vi "Read UUT_Pedigree.vi"(8 "error in (no error)":errorcluster, 11 "Instruments in":refnum<class "Instruments.lvclass">) -> (0 "error out":errorcluster, 2 "Pedigree":enum16{"STAT", "BB", "PT", "EM", "FT"}(ring), 3 "Instruments out":refnum<class "Instruments.lvclass">)   [LabVIEW 2019, in "Instruments.lvlib" / "Instruments.lvclass"]
uses:
  Library/Instruments.lvclass
  Library/Instruments.lvclass/Instruments.ctl
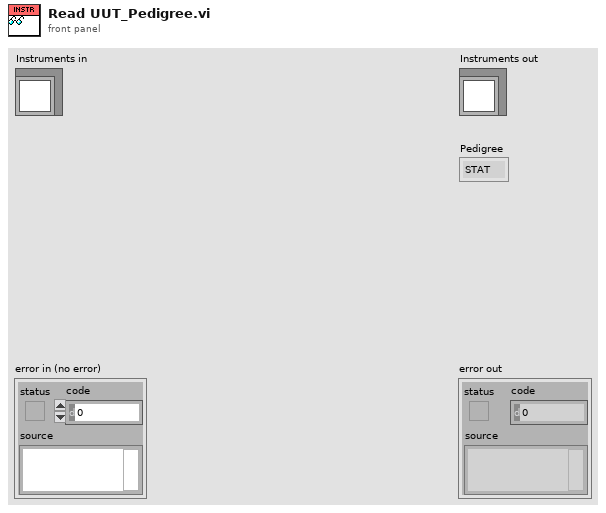
[diagram p1: front panel]
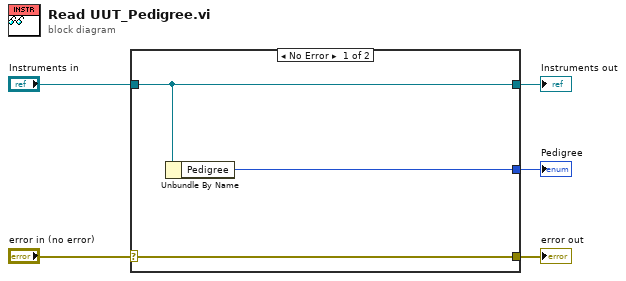
[diagram p0: block diagram]
diagram:
  n1 = case shown="No Error" "error in (no error)" {
    selector: "error in (no error)" -> [w8 w9]
    tunnel: [w8 w9] -> w4
    tunnel: [w7 w10] -> w2
    tunnel: "Instruments in" -> [w7 w10]
    tunnel: [w6 _] -> w1
    frame No Error {
      n2 = Unbundle By Name(w7) -> ("Pedigree"=w6:enum16{"STAT", "BB", "PT", "EM", "FT"})
    }
    frame Error {
    }
  }
  "error out" <- w4
  "Instruments out" <- w2
  "Pedigree" <- w1
